vi "READ ALL TCS ORNL Ver1.vi"() -> ()   [LabVIEW 2016]
uses:
  <vilib>/Platform/TimedLoop/XDataNode/timing_clust.ctl
  <vilib>/Platform/TimedLoop/XDataNode/nitl_modes.ctl
  <vilib>/Platform/TimedLoop/XDataNode/wakeup.ctl
  <vilib>/DAQmx/read.llb/DAQmx Read (Analog 1D DBL NChan 1Samp).vi
  <vilib>/DAQmx/miscellaneous.llb/DAQmx Fill In Error Info.vi
  <vilib>/platform/TimedLoop/XDataNode/XDataNode.xnode
  <vilib>/Platform/TimedLoop/XDataNode/XDNodeRunTimeDep.lvlib
panel:
  out "TC Values":dbl[](array[numeric]) format="%0.2f"
  out "TC Active?":T1
  in  "stop":bool
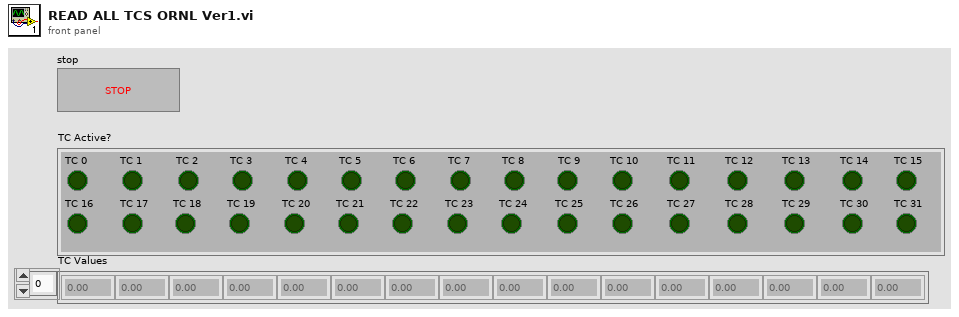
[diagram p1: front panel]
types:
  T1 = cluster{"TC 0":bool, "TC 1":bool, "TC 2":bool, "TC 3":bool, "TC 4":bool, "TC 5":bool, "TC 6":bool, "TC 7":bool, "TC 8":bool, "TC 9":bool, "TC 10":bool, "TC 11":bool, "TC 12":bool, "TC 13":bool, "TC 14":bool, "TC 15":bool, "TC 16":bool, "TC 17":bool, "TC 18":bool, "TC 19":bool, "TC 20":bool, "TC 21":bool, "TC 22":bool, "TC 23":bool, "TC 24":bool, "TC 25":bool, "TC 26":bool, "TC 27":bool, "TC 28":bool, "TC 29":bool, "TC 30":bool, "TC 31":bool}
  T2 = typedef "XDNodeRunTimeDep.lvlib/timing_clust.ctl" = cluster{"Expected End [f-1]":u64, "Actual End [f-1]":u64, "Finished Late? [f-1]":bool, "Expected End [i-1]":u64, "Actual End [i-1]":u64, "Finished Late? [i-1]":bool, "Expected Start [i]":u64, "Actual Start [i]":u64, "Expected Start [f]":u64, "Actual Start [f]":u64, "Source Name":string, "Structure Name":string, "Period":i64, "Deadline":i64, "Offset":i64, "Start":i64, "Priority":i32, "Timeout":i32, "Mode":T3, "Wakeup Reason":T4, "Error":errorcluster, "Source Type":string, "Secondary Source Type":string, "Global End Time":u64, "Global Start Time":u64, "Frame Duration":u64, "Iteration Duration":u64, "Assigned CPU":i32, "I/O Scan Engine Mode":u32}
  T3 = typedef "XDNodeRunTimeDep.lvlib/nitl_modes.ctl" = enum32{"No Change", "Process missed periods, maintain original phase", "Discard missed periods, maintain original phase", "Process missed periods, ignore original phase", "Discard missed periods, ignore original phase"}
  T4 = typedef "XDNodeRunTimeDep.lvlib/wakeup.ctl" = enum32{"Normal", "Aborted", "Asynchronous wakeup", "Timing source error", "Timed loop error", "Timeout"}
  T5 = cluster{"[0]":bool, "[1]":bool, "[2]":bool, "[3]":bool, "[4]":bool, "[5]":bool, "[6]":bool, "[7]":bool, "[8]":bool, "[9]":bool, "[10]":bool, "[11]":bool, "[12]":bool, "[13]":bool, "[14]":bool, "[15]":bool, "[16]":bool, "[17]":bool, "[18]":bool, "[19]":bool, "[20]":bool, "[21]":bool, "[22]":bool, "[23]":bool, "[24]":bool, "[25]":bool, "[26]":bool, "[27]":bool, "[28]":bool, "[29]":bool, "[30]":bool, "[31]":bool}
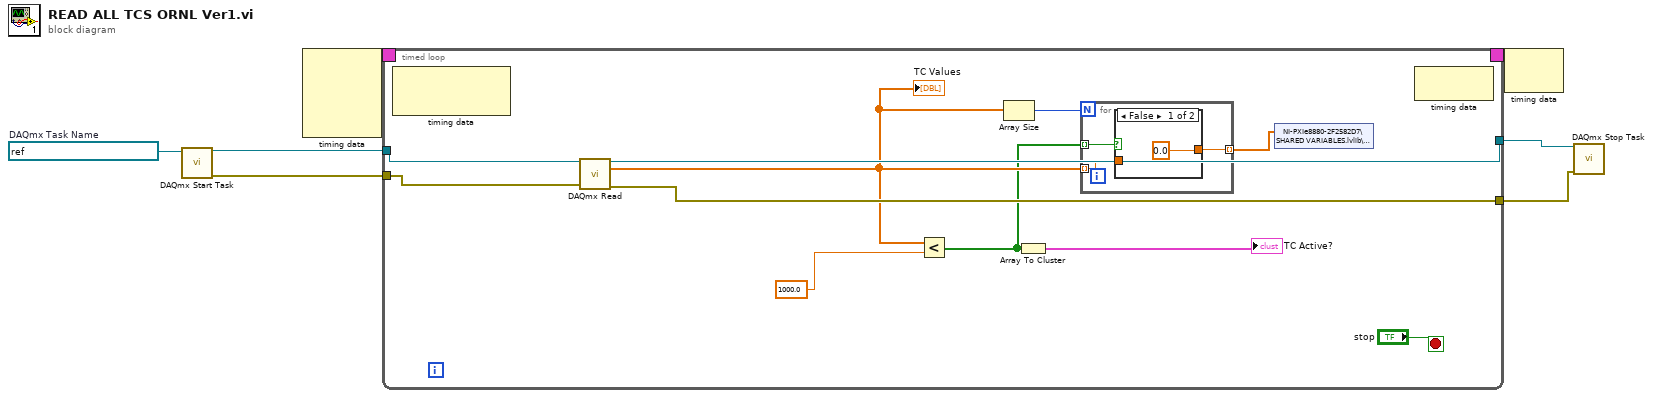
[diagram p0: block diagram]
diagram:
  w7 = refnum<k21> "ALL THERMOCOUPLES"  # DAQmx Task Name
  n1 = call <vilib>:"DAQmx Start Task.vi"("task/channels in"=w7) -> ("task out"=w6:refnum<k21>, "error out"=w4:errorcluster)  [unwired: 13 in]
  n2 = node-c288() -> (w3:T2)  [unwired: 4 in]
  n3 = timed-loop {
    tunnel: w6 -> [w16]
    tunnel: [w16] -> w5
    tunnel: w4 -> [w15]
    timing: w3 -> [_]
    timing-out: [_] -> w2
    tunnel: [w14] -> w1
    stop <- "stop" stop-if-true
    n4 = node-c288() -> ()  [unwired: 1 in, 2 out]
    n5 = call-poly <vilib>:"DAQmx Read.vi"("task/channels in"=w16, "error in"=w15) -> ("data"=w10:dbl[], "error out"=w14:errorcluster)  [unwired: 11 in, 1 out]
    "TC Values" <- w10
    n6 = Less?(x=w10, y=1000.0) -> (x < y?=w9:bool[])
    n7 = Array Size(array=w10) -> (size(s)=w11:i32)
    n8 = Array To Cluster(array=w9) -> (cluster=→"TC Active?":T5)
    n9 = for {
      N: w11 -> [_]
      tunnel: w10 -> [w19] mode=indexing
      tunnel: w9 -> [w20] mode=indexing
      tunnel: [w18] -> w8 mode=indexing
      n10 = case shown="False" w20 {
        tunnel: w19 -> [_ w22]
        tunnel: [0.0 w22] -> w18
        frame False {
        }
        frame True {
        }
      }
    }
    n11 = shared-variable "NI-PXIe8880-2F2582D7\\SHARED VARIABLES.lvlib\\TC's Array"(w8) -> ()  [unwired: 1 in, 1 out]
    n12 = node-c288() -> ()  [unwired: 1 in, 1 out]
  }
  n13 = node-c288(w2) -> ()  [unwired: 1 out]
  n14 = call <vilib>:"DAQmx Stop Task.vi"("task/channels in"=w5, "error in"=w1) -> ()  [unwired: 12 in, 2 out]
